vi "CVCharacterization.vi"() -> ()   [LabVIEW 2020]
panel:
  in  "测量队列":T1(array[cluster])
  out "输出数组":dbl[][](array[numeric])
  out "数据":dbl[][](array[numeric])
  out "XY图":cluster{"序列值":dbl[], dbl[]}[](graph)
  in  "改变量":dbl min=0.0
  in  "分段":dbl[](array[numeric])
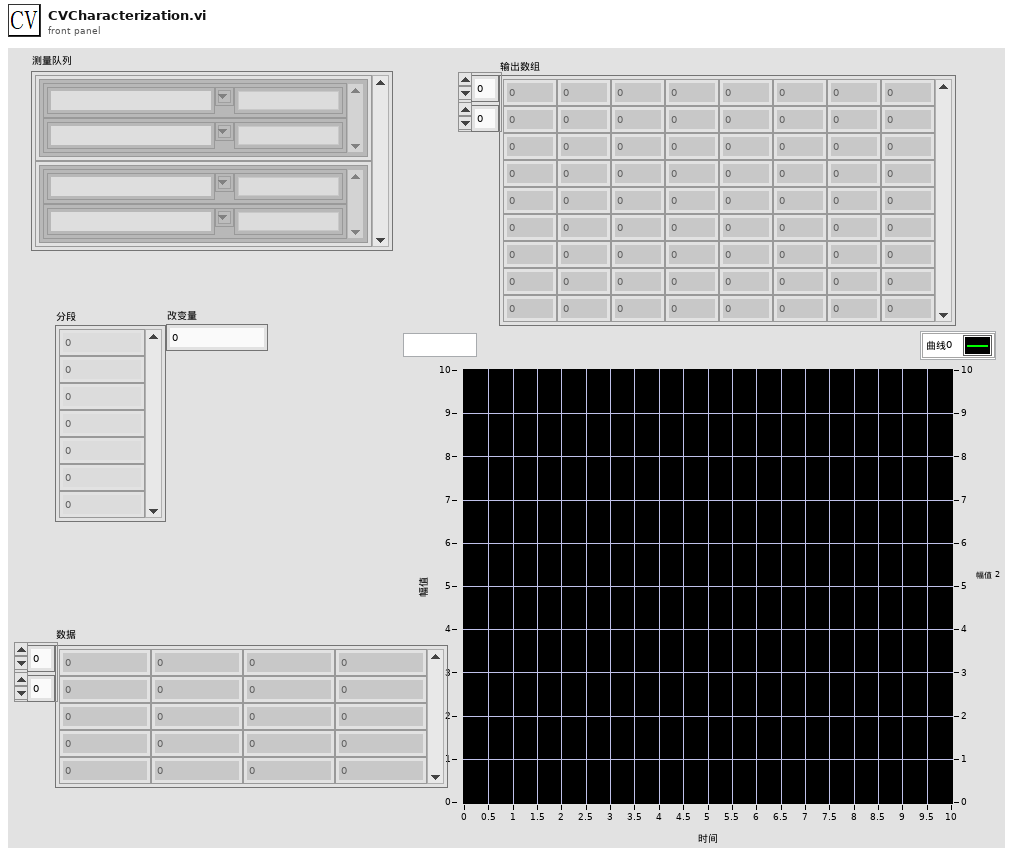
[diagram p1: front panel]
types:
  T1 = cluster{"测量参数":cluster{"设置项":string, "值":string}[]}[]
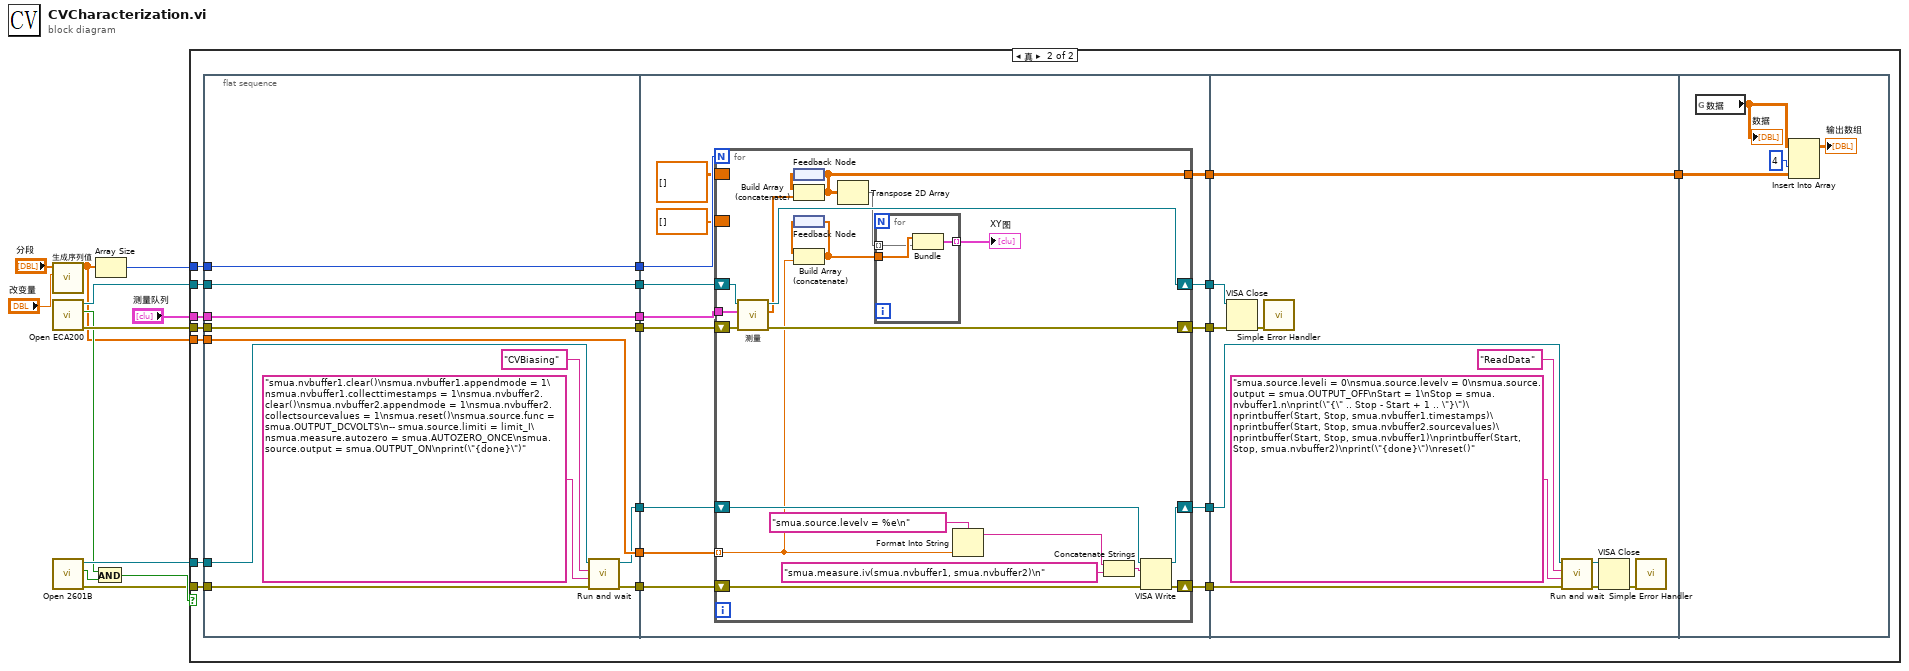
[diagram p0: block diagram]
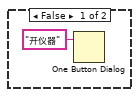
[diagram p2: hidden frame]
diagram:
  n1 = call "生成序列值.vi"("改变量"="改变量", "分段"="分段") -> ("序列值"=w2:dbl[])  [unwired: 9 in]
  n2 = call "Open ECA200.vi"() -> ("错误输出"=w10:errorcluster, "仪器存在"=w4:bool, "VISA资源名称输出"=w11:refnum<visa-resource-name>)  [unwired: 9 in]
  n3 = call "Open 2601B.vi"() -> ("错误输出"=w8:errorcluster, "仪器存在"=w3:bool, "VISA资源名称输出"=w9:refnum<visa-resource-name>)  [unwired: 9 in]
  n4 = And(x=w4, y=w3) -> (x .and. y?=w12:bool)
  n5 = Array Size(array=w2) -> (size(s)=w5:i32)
  n6 = case shown="真" w12 {
    tunnel: w11 -> [_ w33]
    tunnel: w10 -> [_ w32]
    tunnel: w9 -> [_ w20]
    tunnel: w8 -> [_ w21]
    tunnel: w5 -> [_ w31]
    tunnel: w2 -> [_ w30]
    tunnel: "测量队列" -> [_ w29]
    frame False {
      n7 = One Button Dialog(message="开仪器" ("消息")) -> ()  [unwired: 1 in, 1 out]
    }
    frame True {
      n8 = flat-sequence {
        tunnel: w29 -> [w40]
        tunnel: w30 -> [w41]
        tunnel: w31 -> [w42]
        tunnel: w32 -> [w43]
        tunnel: w33 -> [w44]
        tunnel: [w44] -> w28
        tunnel: [w43] -> w27
        tunnel: [w36] -> w26
        tunnel: [w37] -> w25
        tunnel: [w42] -> w24
        tunnel: [w41] -> w23
        tunnel: [w40] -> w22
        tunnel: w21 -> [w39]
        tunnel: w20 -> [w38]
        tunnel: w28 -> [w56]
        tunnel: w27 -> [w55]
        tunnel: w26 -> [w54]
        tunnel: w25 -> [w53]
        tunnel: w24 -> [w52]
        tunnel: w23 -> [w51]
        tunnel: w22 -> [w46]
        tunnel: [w58] -> w19
        tunnel: [w57] -> w18
        tunnel: [w50] -> w17
        tunnel: [w49] -> w16
        tunnel: [w45] -> w15
        tunnel: w19 -> [w90]
        tunnel: w18 -> [w91]
        tunnel: w17 -> [w86]
        tunnel: w16 -> [w85]
        tunnel: w15 -> [w93]
        tunnel: [w93] -> w14
        tunnel: w14 -> [w94]
        frame #0 {
          n9 = call "Run and wait.vi"("错误输入"=w39, "Script"="smua.nvbuffer1.clear()\nsmua.nvbuffer1.appendmode = 1\nsmua.nvbuffer1.collecttimestamps = 1\nsmua.nvbuffer2.clear()\nsmua.nvbuffer2.appendmode = 1\nsmua.nvbuffer2.collectsourcevalues = 1\nsmua.reset()\nsmua.source.func = smua.OUTPUT_DCVOLTS\n-- smua.source.limiti = limit_I\nsmua.measure.autozero = smua.AUTOZERO_ONCE\nsmua.source.output = smua.OUTPUT_ON\nprint(\"{done}\")", "Script Name"="CVBiasing", "VISA资源名称"=w38) -> ("错误输出"=w37:errorcluster, "VISA资源名称输出"=w36:refnum<visa-resource-name>)  [unwired: 6 in]
        }
        frame #1 {
          n10 = for {
            N: w52 -> [_]
            shift-right: [w79] -> w58
            shift-left: w56 -> [w77]
            shift-right: [w78] -> w57
            shift-left: w55 -> [w76]
            shift-right: [w73] -> w49
            shift-left: w54 -> [w75]
            shift-right: [w72] -> w50
            shift-left: w53 -> [w74]
            tunnel: w51 -> [w63] mode=indexing
            border: dbl[][] [] -> [_]
            border: dbl[] [] -> [_]
            tunnel: [w60] -> w45
            tunnel: w46 -> [w59]
            n11 = call "测量.vi"("错误输入（无错误）"=w76, "测量队列"=w59, "VISA资源名称"=w77) -> ("错误输出"=w78:errorcluster, "数组"=w65:dbl[], "VISA资源名称输出"=w79:refnum<visa-resource-name>)  [unwired: 6 in]
            n12 = feedback #1() -> (w66:dbl[][])
            n13 = Build Array (concatenate)(w66, w65) -> (w60:dbl[][])
            n14 = feedback-in #1(w60) -> ()
            n15 = feedback #2() -> (w64:dbl[])
            n16 = Build Array (concatenate)(w64, w63) -> (w61:dbl[])
            n17 = feedback-in #2(w61) -> ()
            n18 = Transpose 2D Array(2D array=w60) -> (transposed array=w62:dbl[][])
            n19 = for {
              tunnel: w62 -> [w81] mode=indexing
              tunnel: w61 -> [w82]
              tunnel: [w80] -> w67 mode=indexing
              n20 = Bundle(w82, w81) -> (w80:cluster{dbl[], dbl[]})  [unwired: 1 in]
            }
            "XY图" <- w67
            n21 = Format Into String(format string="smua.source.levelv = %e\n" ("写入缓冲区"), w63) -> (resulting string=w69:string)  [unwired: 2 in, 1 out]
            n22 = Concatenate Strings(w69, "smua.measure.iv(smua.nvbuffer1, smua.nvbuffer2)\n" ("字符串")) -> (w68:string)
            n23 = VISA Write(VISA resource name=w75, write buffer=w68, error in (no error)=w74) -> (VISA resource name out=w73:refnum<visa-resource-name>, error out=w72:errorcluster)  [unwired: 1 out]
          }
        }
        frame #2 {
          n24 = VISA Close(VISA resource name=w90, error in (no error)=w91) -> (error out=w92:errorcluster)
          n25 = call <vilib>:"Simple Error Handler.vi"("error in (no error)"=w92) -> ()  [unwired: 4 in, 5 out]
          n26 = call "Run and wait.vi"("错误输入"=w86, "Script"="smua.source.leveli = 0\nsmua.source.levelv = 0\nsmua.source.output = smua.OUTPUT_OFF\nStart = 1\nStop = smua.nvbuffer1.n\nprint(\"{\" .. Stop - Start + 1 .. \"}\")\nprintbuffer(Start, Stop, smua.nvbuffer1.timestamps)\nprintbuffer(Start, Stop, smua.nvbuffer2.sourcevalues)\nprintbuffer(Start, Stop, smua.nvbuffer1)\nprintbuffer(Start, Stop, smua.nvbuffer2)\nprint(\"{done}\")\nreset()", "Script Name"="ReadData", "VISA资源名称"=w85) -> ("错误输出"=w89:errorcluster, "VISA资源名称输出"=w88:refnum<visa-resource-name>)  [unwired: 6 in]
          n27 = VISA Close(VISA resource name=w88, error in (no error)=w89) -> (error out=w87:errorcluster)
          n28 = call <vilib>:"Simple Error Handler.vi"("error in (no error)"=w87) -> ()  [unwired: 4 in, 5 out]
        }
        frame #3 {
          n29 = global read "Global variable.vi" "数据"() -> (w97:dbl[][])
          "数据" <- w97
          n30 = Insert Into Array(array=w97, index (col)=4 ("禁用的索引 (列)"), new element=w94) -> (→"输出数组":dbl[][])  [unwired: 1 in]
        }
      }
    }
  }
